vi "test - uuid unique.vi"(8 "error in (no error)":errorcluster, 11 "TestCase in":refnum<class "testcase-Basic-Function.lvclass">) -> (0 "error out":errorcluster, 3 "TestCase out":refnum<class "testcase-Basic-Function.lvclass">)   [LabVIEW 2017, in "testcase-Basic-Function.lvclass"]
uses:
  testcase-Basic-Function.lvclass
  <vilib>/addons/_JKI Toolkits/VI Tester/TestCase.llb/TestCase.lvclass
  src/user.lib/_NEVSTOP/Communicable State Machine(CSM)/Communicable State Machine.lvlib
  C:/Program Files (x86)/National Instruments/LabVIEW 2017/vi.lib/addons/_JKI Toolkits/VI Tester/TestCase.llb/TestCase.lvclass
panel:
  out "Numeric":i32
  out "x != 0?":bool
  out "Array":string[](array[string])
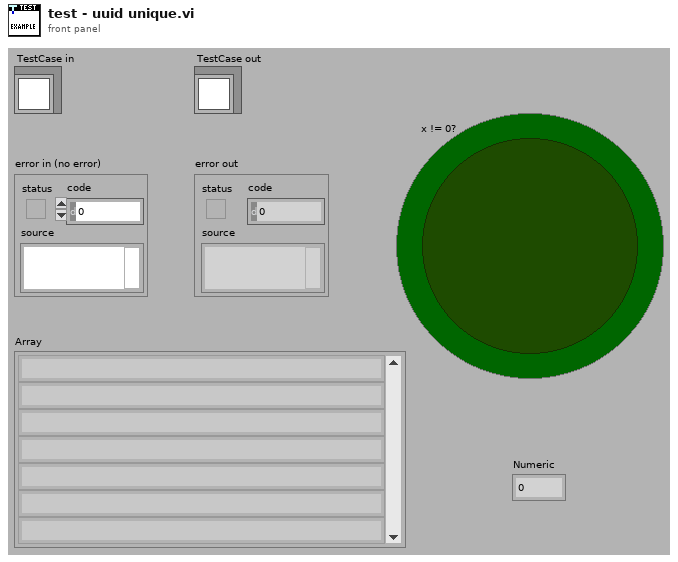
[diagram p1: front panel]
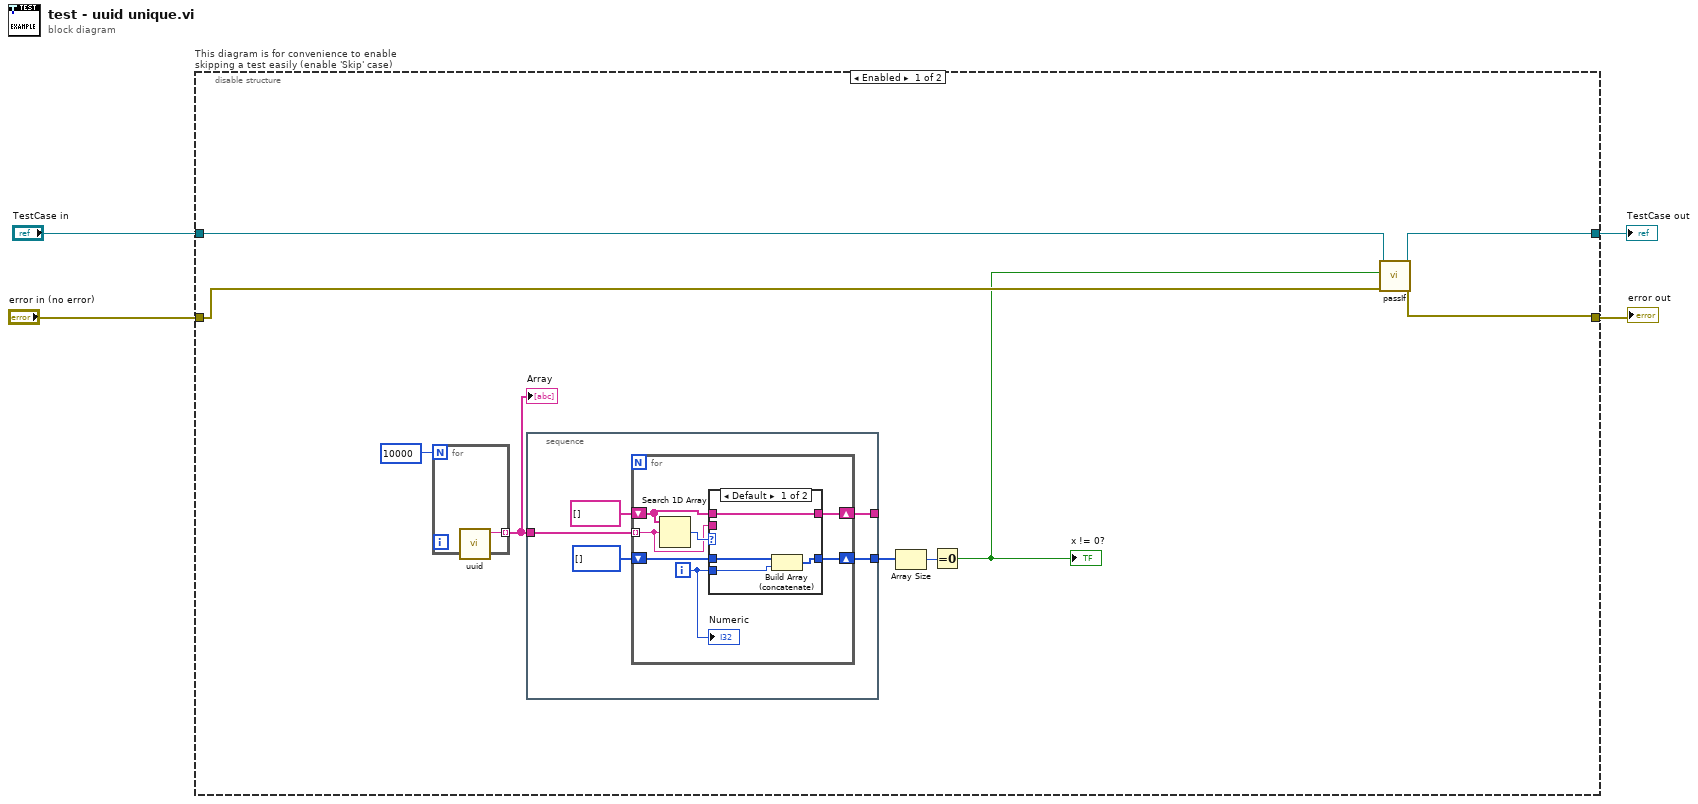
[diagram p0: block diagram]
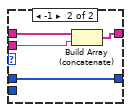
[diagram p2: hidden frame]
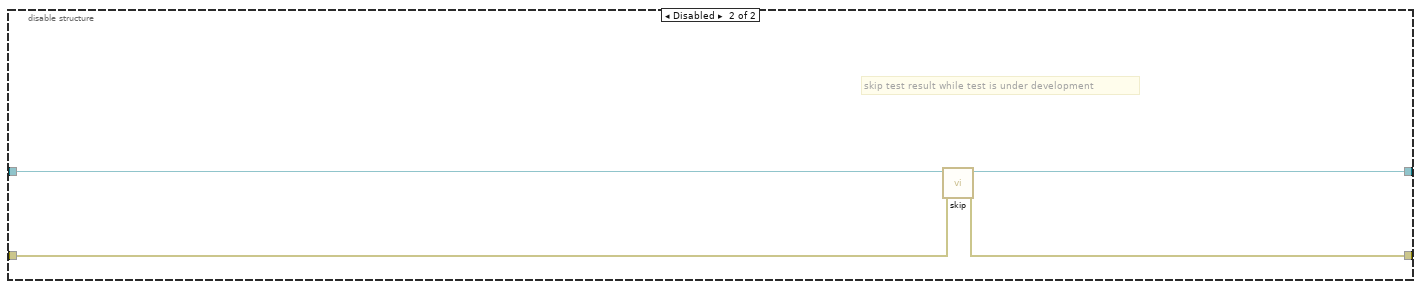
[diagram p3: hidden frame]
diagram:
  n1 = disable-structure "This diagram is for convenience to enable skipping a test easily (enable 'Skip' case)" shown="Enabled" {
    disable-tunnel: "TestCase in" -> [w13 w38]
    disable-tunnel: [w12 w36] -> w1
    disable-tunnel: [w11 w37] -> w3
    disable-tunnel: "error in (no error)" -> [w10 w35]
    frame Enabled {
      n2 = for {
        N: 10000 -> [_]
        tunnel: [w34] -> w8 mode=indexing
        n3 = call "uuid.vi"() -> ("UUID"=w34:string)  [unwired: 11 in]
      }
      "Array" <- w8
      n4 = stacked-sequence {
        tunnel: w8 -> [w14]
        tunnel: [w16] -> _
        tunnel: [w18] -> w7
        frame #0 {
          n5 = for {
            tunnel: w14 -> [w24] mode=indexing
            shift-right: [w23] -> w16
            shift-left: string[] [] -> [w22]
            shift-right: [w20] -> w18
            shift-left: i32[] [] -> [w19]
            i -> [w21]
            n6 = Search 1D Array(1D array=w22, element=w24) -> (index of element=w25:i32)  [unwired: 1 in]
            n7 = case shown="Default" w25 {
              tunnel: w24 -> [_ w33]
              tunnel: [w29 w31] -> w23
              tunnel: w22 -> [w29 w32]
              tunnel: w21 -> [w26 _]
              tunnel: [w27 w30] -> w20
              tunnel: w19 -> [w28 w30]
              frame Default {
                n8 = Build Array (concatenate)(w28, w26) -> (w27:i32[])
              }
              frame -1 {
                n9 = Build Array (concatenate)(w32, w33) -> (w31:string[])
              }
            }
            "Numeric" <- w21
          }
        }
      }
      n10 = Array Size(array=w7) -> (size(s)=w6:i32)
      n11 = Equal To 0?(x=w6) -> (x = 0?=w5:bool)
      "x != 0?" <- w5
      n12 = call-dynamic "passIf.vi"("error in (no error)"=w10, "pass"=w5, "TestCase in"=w13) -> ("error out"=w11:errorcluster, "TestCase out"=w12:refnum<class "testcase-Basic-Function.lvclass">)  [unwired: 7 in]
    }
    frame Disabled {
      # "skip test result while test is under development"
      n13 = call <vilib>:"skip.vi"("error in (no error)"=w35, "TestCase in"=w38) -> ("error out"=w37:errorcluster, "TestCase out"=w36:refnum<class "testcase-Basic-Function.lvclass">)  [unwired: 8 in]
    }
  }
  "error out" <- w3
  "TestCase out" <- w1
